vi "One button pneumatic example.vi"() -> ()   [LabVIEW 2014]
panel:
  out "Output 1":bool
  out "Output 2":bool
  in  "Input 1":bool
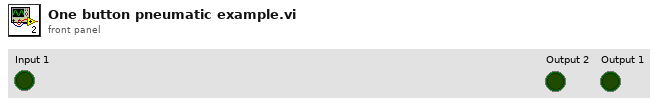
[diagram p1: front panel]
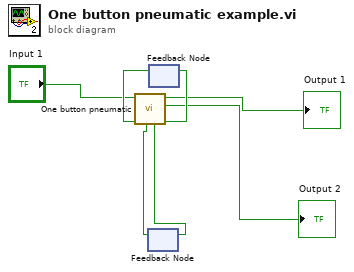
[diagram p0: block diagram]
diagram:
  n1 = feedback #1() -> (w1:bool)  [unwired: 1 in]
  n2 = feedback #2() -> (w6:bool)  [unwired: 1 in]
  n3 = call "One button pneumatic.vi"("Prev State In"=w1, "State In"=w6, "Input 1"="Input 1") -> ("State Out"=w7:bool, "Output 2"=→"Output 2":bool, "Output 1"=→"Output 1":bool, "Prev State Out"=w2:bool)  [unwired: 5 in]
  n4 = feedback-in #1(w2) -> ()
  n5 = feedback-in #2(w7) -> ()
